vi "ex7_1.vi"(10 "Reset Timer":bool) -> (2 "Elapsed Time [ms]":dbl)   [LabVIEW 2022 SP3]
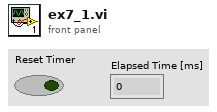
[diagram p1: front panel]
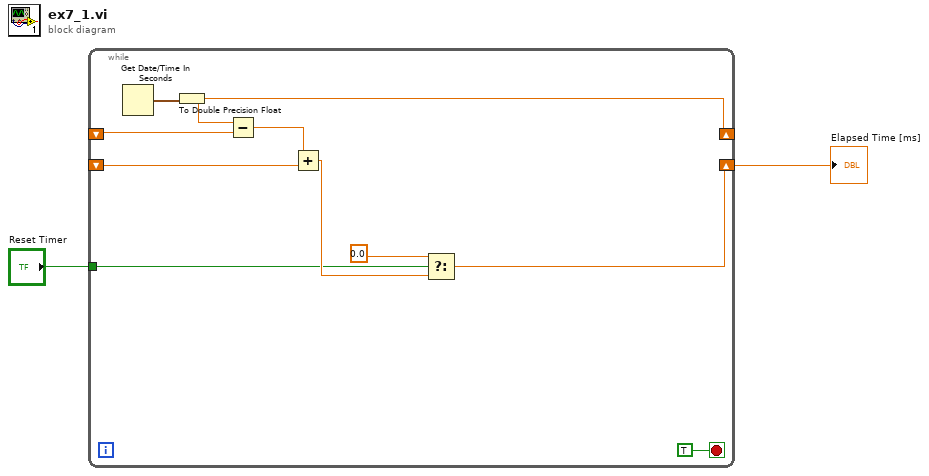
[diagram p0: block diagram]
diagram:
  n1 = while {
    shift-right: [w11] -> _
    shift-left: _ -> [w10]
    shift-right: [w4] -> w1
    shift-left: _ -> [w8]
    tunnel: "Reset Timer" -> [w5]
    stop <- TRUE stop-if-true
    n2 = Get Date/Time In Seconds() -> (seconds since 1Jan1904=w12:timestamp)
    n3 = To Double Precision Float(number=w12) -> (double precision float=w11:dbl)
    n4 = Subtract(x=w11, y=w10) -> (x-y=w9:dbl)
    n5 = Add(x=w9, y=w8) -> (x+y=w7:dbl)
    n6 = Select(t=0.0, s=w5, f=w7) -> (s? t:f=w4:dbl)
  }
  "Elapsed Time [ms]" <- w1
